vi "HandeObj.vi"(0 "reference in":refnum<class "Logger.lvclass">, 11 "error in (no error)":errorcluster) -> (4 "reference out":refnum<class "Logger.lvclass">, 14 "dt":u32, 15 "error out":errorcluster)   [LabVIEW 2019, in "Logger.lvclass"]
uses:
  Logger.lvclass
  Logger.lvclass/Logger.ctl
  2f3f98d4-cfb0-4f81-b92a-0d178dd61f1e.vi
  1c0d0c3d-5d6b-42fa-8895-123650284108.vi
  DatabaseInterface_class/DatabaseInterface.lvclass
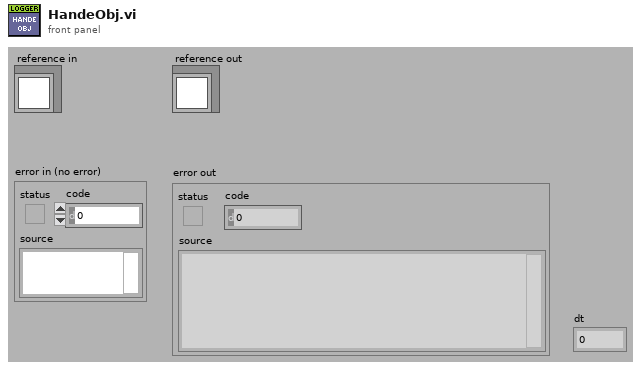
[diagram p1: front panel]
types:
  T1 = typedef "Logger.lvclass/ObjData.ctl" = cluster{"object_tag":string, "parent_tag":string, "object_type":T2, "description":string}
  T2 = typedef "Logger.lvclass/ObjType.ctl" = enum16{"Procces", "Device", "Signal", "DI", "DO", "DA", "AI", "AO", "AA"}
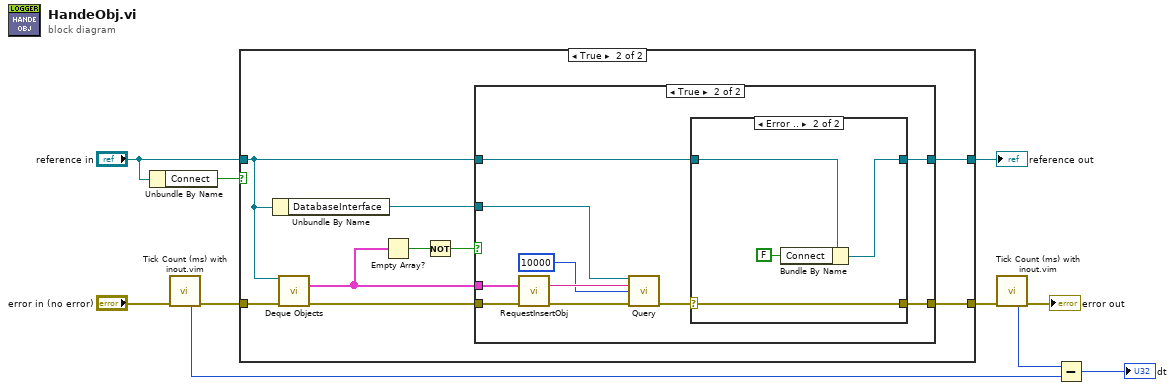
[diagram p0: block diagram]
diagram:
  n1 = Unbundle By Name("reference in") -> ("Connect"=w4:bool)
  n2 = call "Tick Count (ms) with inout.vim"("in"="error in (no error)") -> ("millisecond timer value dub"=w7:u32, "out"=w1:errorcluster)  [unwired: 12 in, 1 out]
  n3 = case shown="True" w4 {
    tunnel: [w12 w21] -> w5
    tunnel: w1 -> [w12 w16]
    tunnel: "reference in" -> [w11 w17]
    tunnel: [w11 w18] -> w3
    frame False {
    }
    frame True {
      n4 = Unbundle By Name(w17) -> ("DatabaseInterface"=w19:refnum<class "DatabaseInterface.lvclass">)
      n5 = call "Deque Objects.vi"("reference in"=w17, "error in (no error)"=w16) -> ("remaining elements"=w14:T1[], "error out"=w15:errorcluster)  [unwired: 12 in]
      n6 = Empty Array?(array=w14) -> (empty?=w20:bool)
      n7 = Not(x=w20) -> (.not. x?=w13:bool)
      n8 = case shown="True" w13 {
        tunnel: w15 -> [w23 w33]
        tunnel: w19 -> [_ w30]
        tunnel: [w23 w26] -> w21
        tunnel: w14 -> [_ w28]
        tunnel: w17 -> [w22 w25]
        tunnel: [w22 w24] -> w18
        frame False {
        }
        frame True {
          n9 = call "RequestInsertObj.vi"("Array"=w28, "error in (no error)"=w33) -> ("request"=w31:string, "error out"=w32:errorcluster)  [unwired: 12 in]
          n10 = call-dynamic "Query.vi"("reference in"=w30, "Query"=w31, "Timeout"=10000, "error in (no error)"=w32) -> ("error out"=w27:errorcluster)  [unwired: 9 in, 2 out]
          n11 = case shown="Error .." w27 {
            selector: w27 -> [w35 w39]
            tunnel: [w35 w39] -> w26
            tunnel: w25 -> [w34 w38]
            tunnel: [w34 w36] -> w24
            frame No Error {
            }
            frame Error {
              n12 = Bundle By Name(cluster=w38, "Connect"=FALSE) -> (w36:refnum<class "Logger.lvclass">)
            }
          }
        }
      }
    }
  }
  "reference out" <- w3
  n13 = call "Tick Count (ms) with inout.vim"("in"=w5) -> ("millisecond timer value dub"=w8:u32, "out"=→"error out":errorcluster)  [unwired: 12 in, 1 out]
  n14 = Subtract(x=w8, y=w7) -> (x-y=→"dt":u32)
